vi "table2bd.vi"(3 "error in (no error)":errorcluster, 4 "eeert":string[][](table)=[["", "Фаза", "Ch0", "6", "Градусы"], ["", "Фаза", "Ch1", "7", "Градусы"], ["", "Фаза", "Ch2", "1", "Градусы"], ["", "Фаза", "Ch3", "2", "Градусы"], ["", "Фаза", "Ch4", "3", "Градусы"], ["", "Напряжение/Ток", "Ch0", "0,00", "В"], ["", "Напряжение/Ток", "Ch1", "0,00", "В"], ["", "Напряжение/Ток", "Ch2", "0,00", "В"], ["", "Напряжение/Ток", "Ch3", "0,00", "В"], ["", "Напряжение/Ток", "Ch4", "0,00", "В"], ["", "Частота", "Ch0", "300,00", "Гц"]], 5 "time stamp":timestamp) -> (0 "error out":errorcluster)   [LabVIEW 2010]
uses:
  <vilib>/addons/database/Auxilliary.llb/DB Tools Column Info.ctl
  <vilib>/addons/database/Auxilliary.llb/DB Tools DataTypes.ctl
  70user.lib/TheSigTab.vi
  <vilib>/addons/database/Connection.llb/Conn Execute.vi
  <vilib>/addons/database/NI_Database_API.lvlib
panel:
  out "Array":string[](array[string])
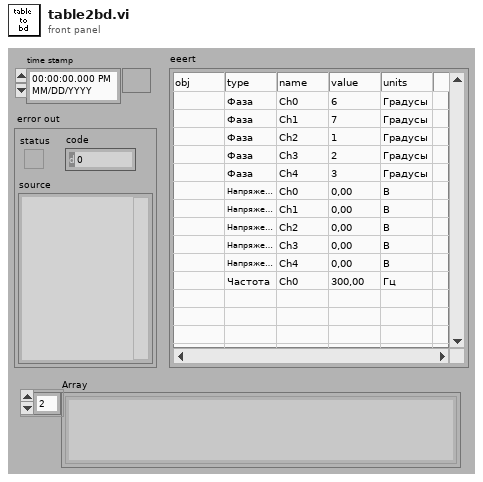
[diagram p1: front panel]
types:
  T1 = cluster{"type":string, "name":string, "val":dbl, "units":string, "sig_id":i32, "date_time":string, "obj_id":i32}
  T2 = typedef "NI_Database_API.lvlib/DB Tools Column Info.ctl" = cluster{"column name":string, "data type":T3, "size":i32, "allow null?":bool}
  T3 = typedef "NI_Database_API.lvlib/DB Tools DataTypes.ctl" = enum16{"String", "Long (I32)", "Single (SGL)", "Double (DBL)", "Date/Time", "Binary"}
  T4 = typedef "NI_Database_API.lvlib/Conn ObjectReference.ctl" = refnum<k1>
  T5 = cluster{"eeert[0]":string, "eeert[1]":string, "eeert[2]":string, "eeert[3]":string, "eeert[4]":string}
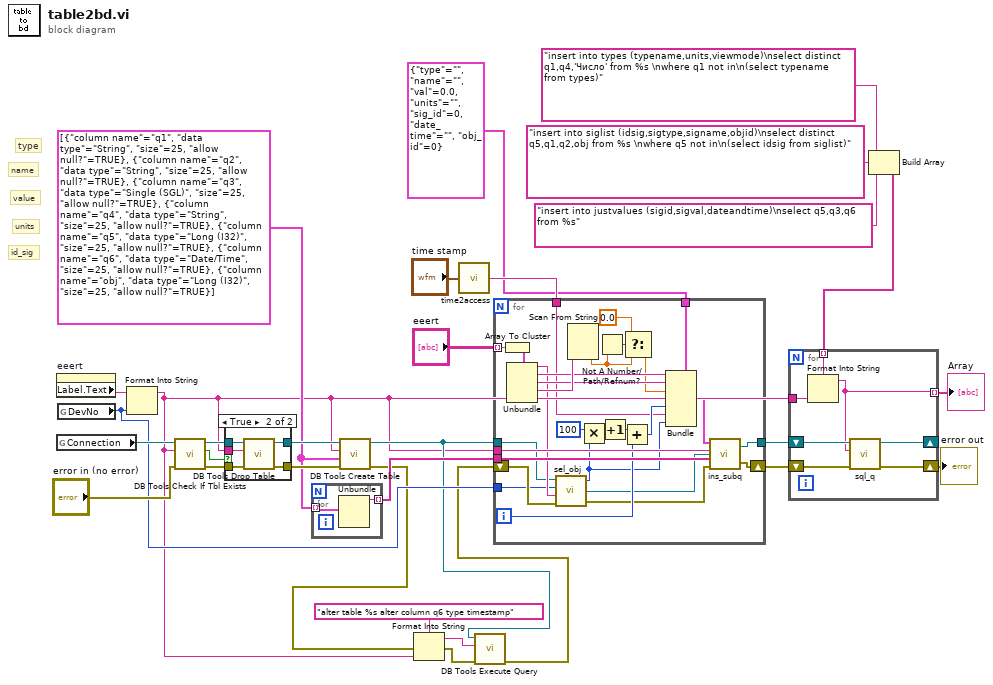
[diagram p0: block diagram]
diagram:
  w26 = T2[] [{"column name"="q1", "data type"=enum."String", "size"=25, "allow null?"=TRUE}, {"column name"="q2", "data type"=enum."String", "size"=25, "allow null?"=TRUE}, {"column name"="q3", "data type"=enum."Single (SGL)", "size"=25, "allow null?"=TRUE}, {"column name"="q4", "data type"=enum."String", "size"=25, "allow null?"=TRUE}, {"column name"="q5", "data type"=enum."Long (I32)", "size"=25, "allow null?"=TRUE}, {"column name"="q6", "data type"=enum."Date/Time", "size"=25, "allow null?"=TRUE}, {"column name"="obj", "data type"=enum."Long (I32)", "size"=25, "allow null?"=TRUE}]
  # "value"
  # "name"
  # "id_sig"
  # "units"
  # "type"
  n1 = property on="eeert" class="Tbl (strict)"() -> ("Label.Text"=w25:string)  [unwired: 2 in, 2 out]
  n2 = global read "TheSigTab.vi" "Connection"() -> (w20:T4)
  n3 = global read "TheSigTab.vi" "DevNo"() -> (w10:u32)
  n4 = Format Into String(initial string=w25, w10) -> (resulting string=w2:string)  [unwired: 2 in, 1 out]
  n5 = call <vilib>:"DB Tools Check If Tbl Exists.vi"("error in (no error)"="error in (no error)", "table name"=w2, "connection reference"=w20) -> ("error out"=w21:errorcluster, "exists?"=w23:bool, "connection reference out"=w22:T4)  [unwired: 2 in]
  n6 = case shown="True" w23 {
    tunnel: [w32 w37] -> w30
    tunnel: w2 -> [_ w36]
    tunnel: [w31 w35] -> w29
    tunnel: w22 -> [w32 w34]
    tunnel: w21 -> [w31 w33]
    frame False {
    }
    frame True {
      n7 = call <vilib>:"DB Tools Drop Table.vi"("error in (no error)"=w33, "table"=w36, "connection reference"=w34) -> ("error out"=w35:errorcluster, "connection reference out"=w37:T4)  [unwired: 5 in]
    }
  }
  n8 = for {
    tunnel: w26 -> [w39] mode=indexing
    tunnel: [w38] -> w24 mode=indexing
    n9 = Unbundle(w39) -> ("column name"=w38:string)  [unwired: 3 out]
  }
  n10 = call <vilib>:"DB Tools Create Table.vi"("error in (no error)"=w29, "column information"=w26, "table"=w2, "connection reference"=w30) -> ("error out"=w7:errorcluster, "connection reference out"=w4:T4)  [unwired: 4 in]
  n11 = Format Into String(format string="alter table %s alter column q6 type timestamp", error in=w7, w2) -> (resulting string=w5:string, error out=w6:errorcluster)  [unwired: 1 in]
  n12 = call "time2access.vi"("time stamp"="time stamp") -> ("date/time string"=w28:string)
  n13 = call-poly <vilib>:"DB Tools Execute Query.vi"("error in (no error)"=w6, "SQL query"=w5, "connection reference"=w4) -> ("error out"=w3:errorcluster)  [unwired: 5 in, 1 out]
  n14 = for {
    tunnel: [w67] -> w16
    tunnel: w2 -> [w66]
    tunnel: w4 -> [w54]
    tunnel: w24 -> [w65]
    tunnel: "eeert" -> [w64] mode=indexing
    shift-right: [w68] -> w17
    shift-left: w3 -> [w52]
    tunnel: w28 -> [w47]
    tunnel: w10 -> [w41]
    tunnel: T1 {"type"="", "name"="", "val"=0.0, "units"="", "sig_id"=0, "date_time"="", "obj_id"=0} ("anything") -> [w40]
    i -> [w62]
    n15 = Array To Cluster(array=w64) -> (cluster=w61:T5)
    n16 = Unbundle(w61) -> ("eeert[0]"=w55:string, "eeert[1]"=w56:string, "eeert[2]"=w57:string, "eeert[3]"=w58:string, "eeert[4]"=w59:string)
    n17 = call "sel_obj.vi"("error in"=w52, "Object"=w55, "DevNo"=w41, "conn ref in"=w54) -> ("error out"=w51:errorcluster, "conn ref out"=w53:T4, "Obj Id"=w42:i32)
    n18 = Scan From String(input string=w58) -> (output 1=w45:dbl)  [unwired: 4 in, 3 out]
    n19 = Multiply(x=100, y=w42) -> (x*y=w50:i32)
    n20 = Not A Number/Path/Refnum?(number/path/refnum=w45) -> (NaN/Path/Refnum?=w46:bool)
    n21 = Increment(x=w50) -> (x+1=w48:i32)
    n22 = Add(x=w48, y=w62) -> (x+y=w60:i32)
    n23 = Select(t=0.0, s=w46, f=w45) -> (s? t:f=w43:dbl)
    n24 = Bundle(cluster=w40, "type"=w56, "name"=w57, "val"=w43, "units"=w59, "sig_id"=w60, "date_time"=w47, "obj_id"=w42) -> (w63:T1)
    n25 = call "ins_subq.vi"("data"=w63, "table_name"=w66, "columns"=w65, "error out"=w51, "conn ref out"=w53) -> ("connection reference out"=w67:T4, "error out 2"=w68:errorcluster)
  }
  n26 = Build Array("insert into types (typename,units,viewmode)\nselect distinct q1,q4,'Число' from %s \nwhere q1 not in\n(select typename from types)" ("optional clause"), "insert into siglist (idsig,sigtype,signame,objid)\nselect distinct q5,q1,q2,obj from %s \nwhere q5 not in\n(select idsig from siglist)", "insert into justvalues (sigid,sigval,dateandtime)\nselect q5,q3,q6 from %s") -> (w11:string[])
  n27 = for {
    tunnel: w2 -> [w75]
    shift-right: [w71] -> _
    shift-left: w16 -> [w73]
    shift-right: [w72] -> w12
    shift-left: w17 -> [w74]
    tunnel: w11 -> [w70] mode=indexing
    tunnel: [w69] -> w1 mode=indexing
    n28 = Format Into String(format string=w70, w75) -> (resulting string=w69:string)  [unwired: 2 in, 1 out]
    n29 = call "sql_q.vi"("error in"=w74, "SQL query"=w69, "connect ref"=w73) -> ("error out"=w72:errorcluster, "conn ref out"=w71:T4)  [unwired: 1 in, 2 out]
  }
  "error out" <- w12
  "Array" <- w1
